vi "create-new.vi"(8 "error in (no error)":errorcluster) -> (0 "error out":errorcluster, 3 "UUID out":refnum<class "UUID.lvclass">)   [LabVIEW 2020, in "graph.lvlib" / "UUID.lvclass"]
uses:
  UUID.lvclass
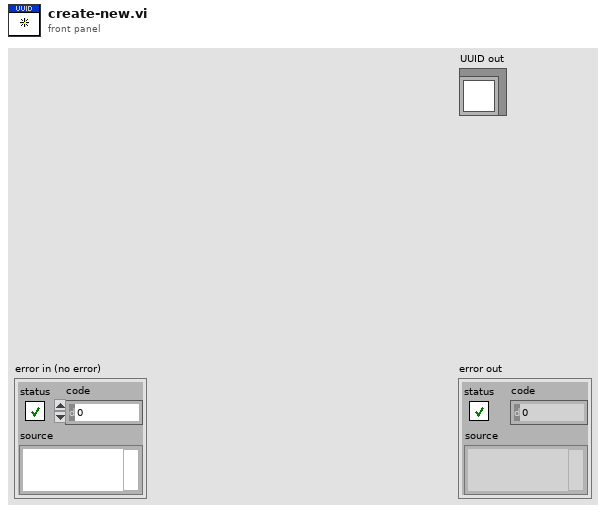
[diagram p1: front panel]
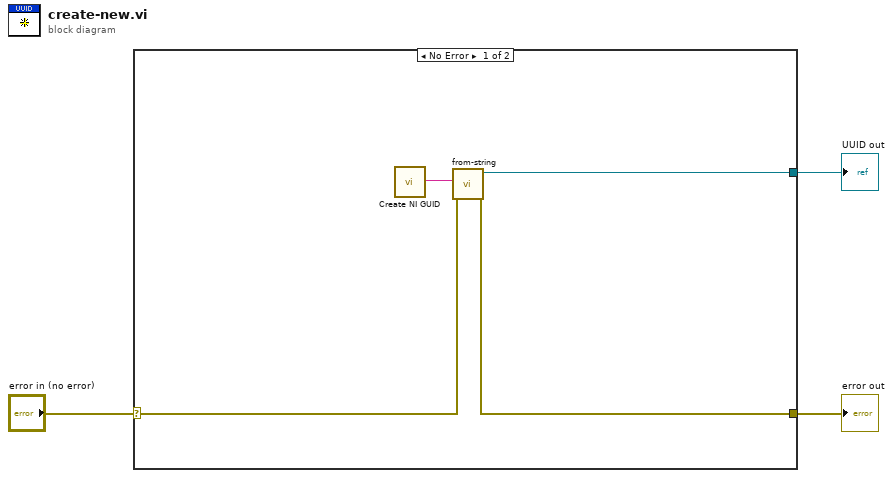
[diagram p0: block diagram]
diagram:
  n1 = case shown="No Error" "error in (no error)" {
    selector: "error in (no error)" -> [w5 w8]
    tunnel: [w4 w8] -> w2
    tunnel: [w6 _] -> w1
    frame No Error {
      n2 = call <vilib>:"Create NI GUID.vi"() -> ("NI GUID"=w7:string)
      n3 = call "from-string.vi"("error in (no error)"=w5, "uuid-string"=w7) -> ("error out"=w4:errorcluster, "UUID out"=w6:refnum<class "UUID.lvclass">)  [unwired: 8 in]
    }
    frame Error {
    }
  }
  "error out" <- w2
  "UUID out" <- w1
